vi "climber_globals.vi"() -> ()   [LabVIEW 2020]
panel:
  out "Climber Lower Command":bool
  out "Climber Raise Command":bool
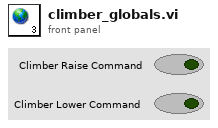
[diagram p1: front panel]
diagram:
